vi "Browse for XNET Database.vi"(8 "error in (no error)":errorcluster) -> (0 "error out":errorcluster, 1 "J1939 Monitor Settings":T1 {"Name" format="%.0x"}, 2 "Cancel Out":bool, 3 "J1939 XNET Settings":T2={"Database"="", "Cluster"="", "Port"="", "Baud rate [Bd]"=0, "Termination"=0, "Incoming Decimation"=0, "Outgoing Decimation"=0, "Async Read Rate"=1, "Async Write Rate"=1} {"Termination" items=["Off", "On"]})   [LabVIEW 2019, in "J1939 Addon System Explorer.lvlib"]
uses:
  J1939 Addon System Explorer.lvlib
  Addon Shared/Types/XNET Settings.ctl
  Addon Shared/Types/Monitor Settings.ctl
  <resource>/objmgr/xnet.rc
  Addon Shared/J1939 Addon Shared.lvlib
panel:
  in  "Name":u64=1 format="%.0x"
  in  "Address":u8 format="%.0x"
  in  "Baud rate [Bd]":u32=500000
  in  "Select CAN Cluster":u16(ring) items=["j1939.Cluster"]
  in  "Cancel":bool
  in  "Select":bool
  in  "XNET Database":refnum<k21>
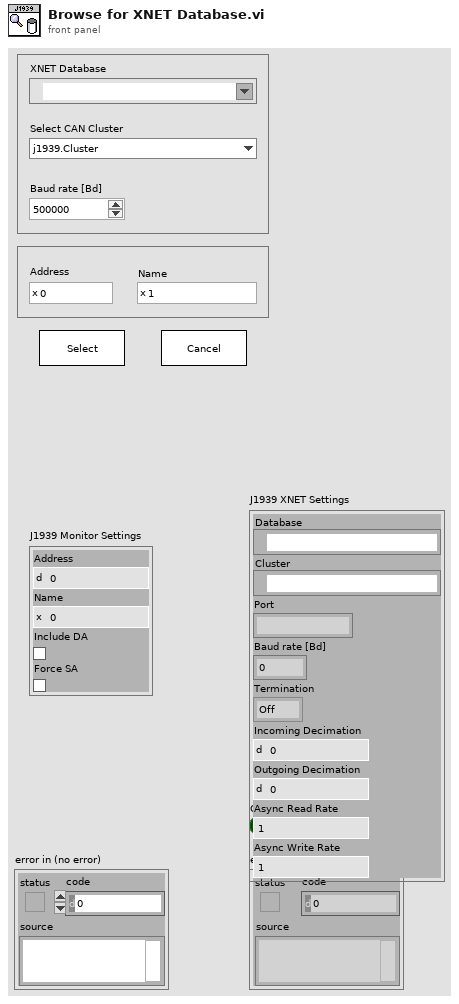
[diagram p1: front panel]
types:
  T1 = typedef "J1939 Addon Shared.lvlib/Monitor Settings.ctl" = cluster{"Address":u8, "Name":u64, "Include DA":bool, "Force SA":bool}
  T2 = typedef "J1939 Addon Shared.lvlib/XNET Settings.ctl" = cluster{"Database":refnum<k21>, "Cluster":refnum<k21>, "Port":string, "Baud rate [Bd]":u32, "Termination":u32, "Incoming Decimation":u32, "Outgoing Decimation":u32, "Async Read Rate":u32, "Async Write Rate":u32}
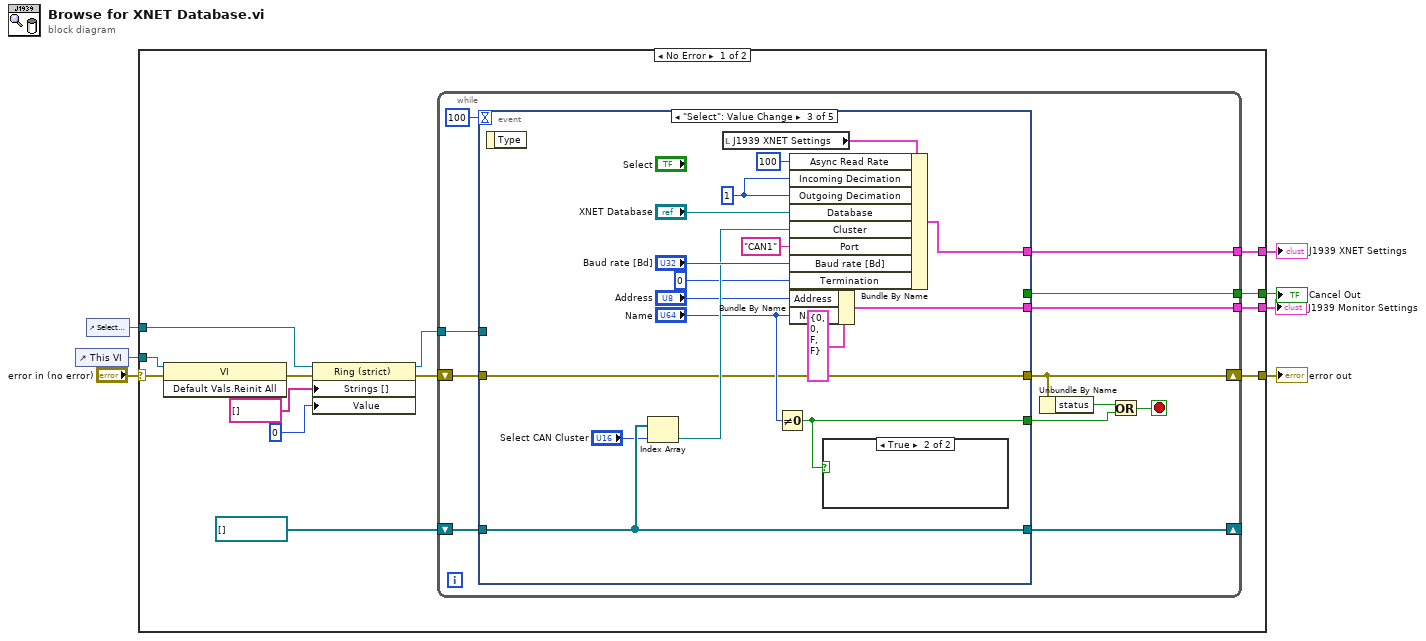
[diagram p0: block diagram]
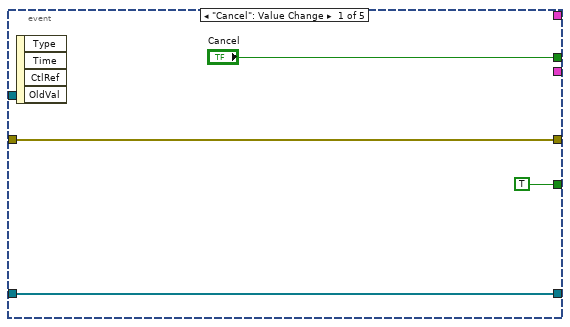
[diagram p2: hidden frame]
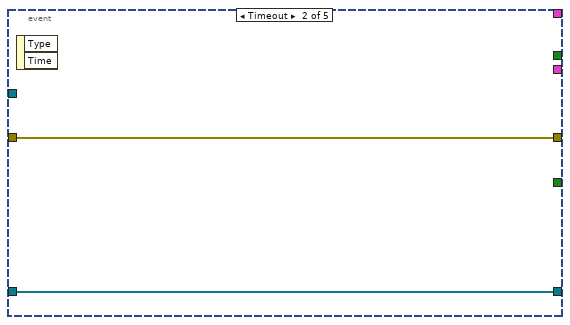
[diagram p3: hidden frame]
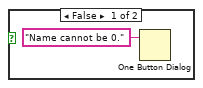
[diagram p4: hidden frame]
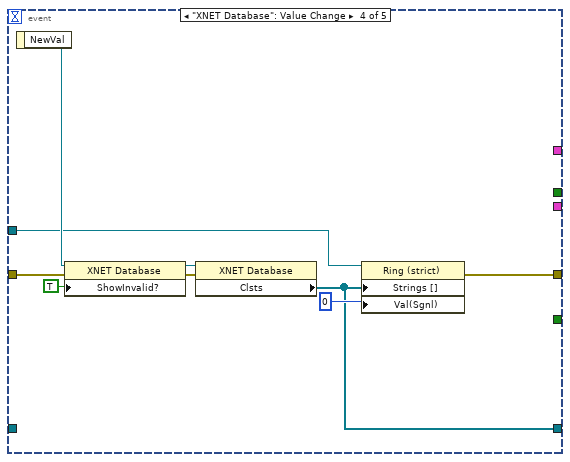
[diagram p5: hidden frame]
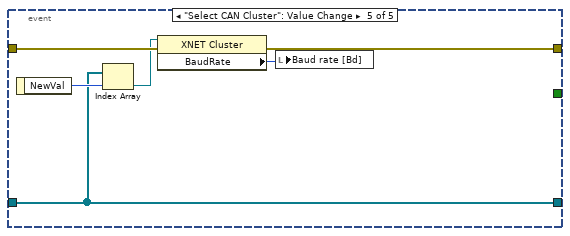
[diagram p6: hidden frame]
diagram:
  n1 = control-ref of="This VI"() -> (w4:refnum<vi>)
  n2 = control-ref of="Select CAN Cluster"() -> (w2:refnum<vi>)
  n3 = case shown="No Error" "error in (no error)" {
    selector: "error in (no error)" -> [w19 w72]
    tunnel: [w17 w72] -> w6
    tunnel: [w20 _] -> w5
    tunnel: w4 -> [w18 _]
    tunnel: [w15 _] -> w3
    tunnel: w2 -> [w14 _]
    tunnel: [w8 _] -> w1
    frame No Error {
      n4 = invoke class="VI" method="Default Vals.Reinit All"(reference=w18, error in=w19) -> (error out=w13:errorcluster)  [unwired: 1 in, 2 out]
      n5 = property on="Property Node" class="Ring (strict)"(reference=w14, error in=w13, "Strings []"=string[] [], "Value"=u16 0) -> (reference out=w12:refnum<vi>, error out=w11:errorcluster)
      n6 = while {
        tunnel: [w32] -> w20
        shift-right: [w30] -> _
        shift-left: refnum<k21>[] [] ("Clsts") -> [w29]
        shift-right: [w26] -> w17
        shift-left: w11 -> [w31]
        tunnel: [w28] -> w15
        tunnel: w12 -> [w22]
        tunnel: [w21] -> w8
        stop <- w23 stop-if-true
        n7 = event shown="[2] \"Select\": Value Change" {
          selector: _ -> [_ _ _ _ _]
          dyn-events: _ -> [_ _ _ _ _]
          timeout: 100 -> [_ _ _ _ _]
          tunnel: ["Cancel" _ _ _ _] -> w32
          tunnel: w31 -> [w34 w38 w41 w62 w70]
          tunnel: [w35 w37 w52 w59 w66] -> w30
          tunnel: w29 -> [w35 w37 w52 _ w66]
          tunnel: [w34 w38 w41 w57 w69] -> w26
          tunnel: [_ _ w49 _ _] -> w28
          tunnel: [TRUE _ w42 _ _] -> w24
          tunnel: w22 -> [_ _ _ w58 _]
          tunnel: [_ _ w45 _ _] -> w21
          event "Cancel": Value Change {
            n8 = event-data() -> ()  [unwired: 1 in, 4 out]
          }
          event Timeout {
            n9 = event-data() -> ()  [unwired: 1 in, 2 out]
          }
          event "Select": Value Change {
            w44 = u32 1 ("Outcoming Rate")
            n10 = event-data() -> ()  [unwired: 1 in, 1 out]
            n11 = Index Array(array=w52, index="Select CAN Cluster") -> (element=w50:refnum<k21>)
            n12 = local read "J1939 XNET Settings"() -> (w53:T2)
            n13 = Not Equal To 0?(x="Name") -> (x != 0?=w42:bool)
            n14 = Bundle By Name(cluster=w53, "Async Read Rate"=u32 100, "Incoming Decimation"=w44, "Outgoing Decimation"=w44, "Database"="XNET Database", "Cluster"=w50, "Port"="CAN1", "Baud rate [Bd]"="Baud rate [Bd]", "Termination"=u32 0) -> (w49:T2)
            n15 = Bundle By Name(cluster=T1 {"Address"=0, "Name"=0, "Include DA"=FALSE, "Force SA"=FALSE} ("J1939 Monitor Settings"), "Address"="Address", "Name"="Name") -> (w45:T1)
            n16 = case shown="True" w42 {
              frame False {
                n17 = One Button Dialog(message="Name cannot be 0.") -> ()  [unwired: 1 in, 1 out]
              }
              frame True {
              }
            }
          }
          event "XNET Database": Value Change {
            n18 = event-data() -> ("NewVal"=w61:refnum<k21>)  [unwired: 1 in]
            n19 = property class="XNET Database"(reference=w61, error in=w62, "ShowInvalid?"=TRUE ("Show Invalid From Open?")) -> (reference out=w65:refnum<k21>, error out=w64:errorcluster)
            n20 = property class="XNET Database"(reference=w65, error in=w64) -> ("Clsts"=w59:refnum<k21>[])  [unwired: 2 out]
            n21 = property on="Property Node" class="Ring (strict)"(reference=w58, "Strings []"=w59, "Val(Sgnl)"=u16 0 ("Value (Signaling)")) -> (error out=w57:errorcluster)  [unwired: 1 in, 1 out]
          }
          event "Select CAN Cluster": Value Change {
            n22 = event-data() -> ("NewVal"=w68:u16)  [unwired: 1 in]
            n23 = Index Array(array=w66, index=w68) -> (element=w67:refnum<k21>)
            n24 = property class="XNET Cluster"(reference=w67, error in=w70) -> (error out=w69:errorcluster, "BaudRate"=w71:u32)  [unwired: 1 out]
            n25 = local write "Baud rate [Bd]"(w71) -> ()
          }
        }
        n26 = Unbundle By Name(w26) -> ("status"=w25:bool)
        n27 = Or(x=w25, y=w24) -> (x .or. y?=w23:bool)
      }
    }
    frame Error {
    }
  }
  "error out" <- w6
  "Cancel Out" <- w5
  "J1939 XNET Settings" <- w3
  "J1939 Monitor Settings" <- w1
